vi "RTE PPL Test.vi"() -> ()   [LabVIEW 2020]
uses:
  PPL/HDH.ProjectBuilder.lvlibp/Class/PPL Class Test/PPL Class Test.lvclass
  PPL/HDH.ProjectBuilder.lvlibp/Class/Project Builder/Project Builder.lvclass
  PPL/HDH.ProjectBuilder.lvlibp/Class/PPL Class Test/PPL Class Test Data/PPL Class Test Data.lvclass
  PPL/HDH.ProjectBuilder.lvlibp/Interface/Action Interface/Action Interface.lvclass
  PPL/HDH.ProjectBuilder.lvlibp
panel:
  out "Load Success":string[](array[string])
  out "Load Failure":string[](array[string])
  out "Success?":bool
  in  "Run":bool
  in  "PPL Name in PPL folder (entire PPL folder if empty)":string
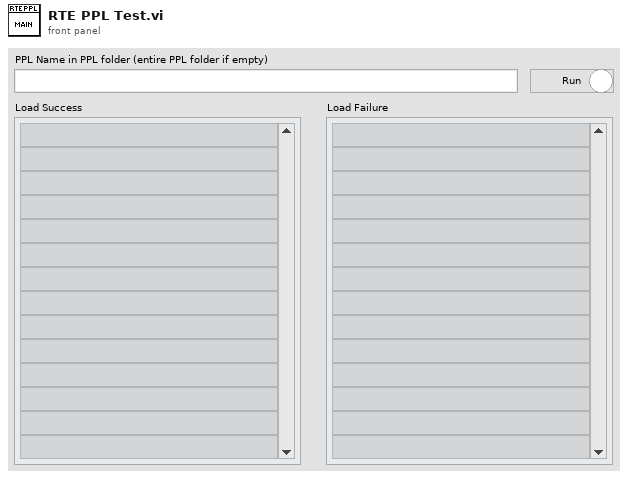
[diagram p1: front panel]
types:
  T1 = enum32{"Invalid", "Standard", "Closed", "Hidden", "Minimized", "Maximized"}
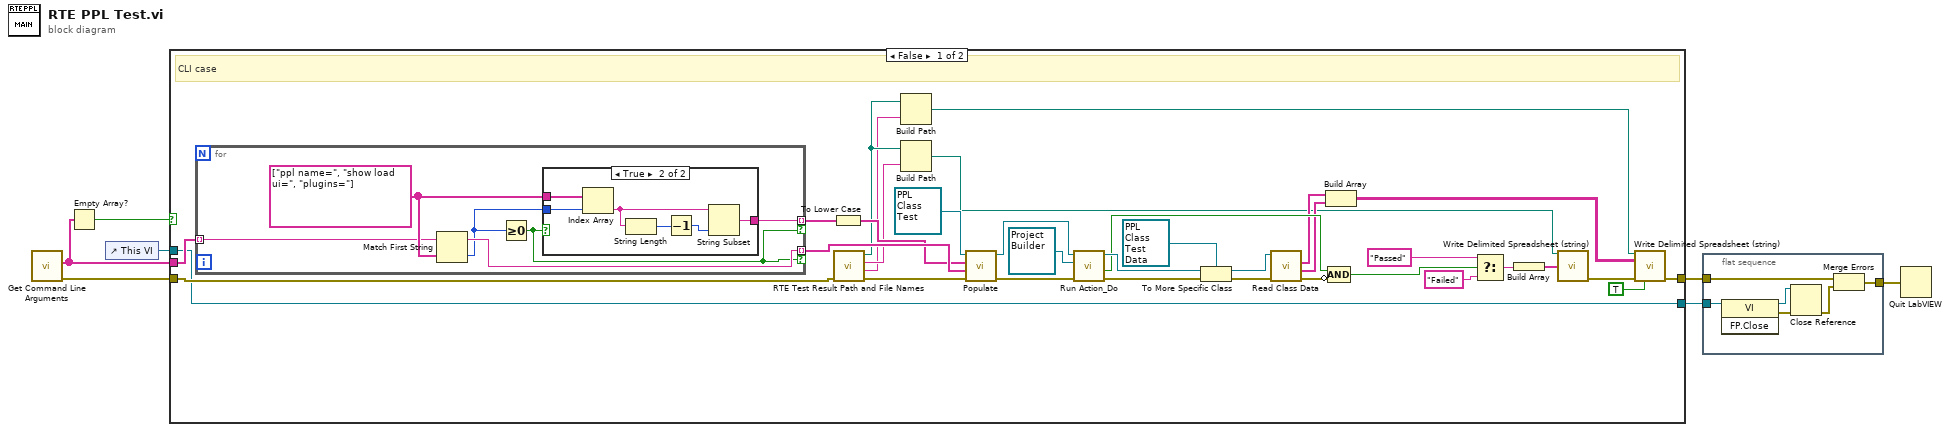
[diagram p0: block diagram]
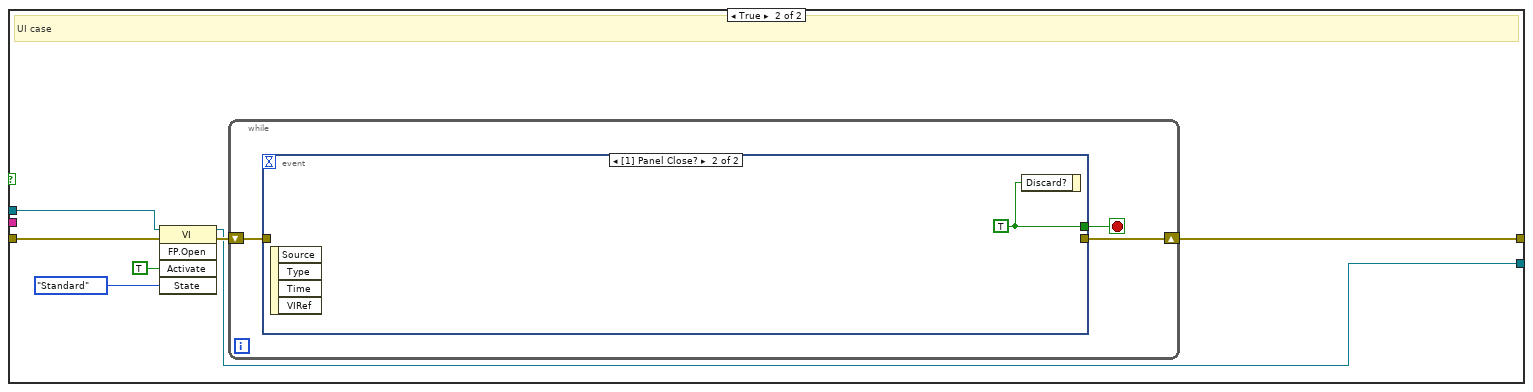
[diagram p3: hidden frame]
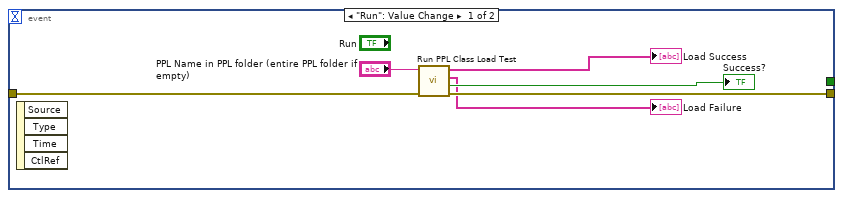
[diagram p4: hidden frame]
diagram:
  n1 = call <vilib>:"Get Command Line Arguments.vi"() -> ("error out"=w5:errorcluster, "arguments"=w6:string[])  [unwired: 9 in, 1 out]
  n2 = Empty Array?(array=w6) -> (empty?=w7:bool)
  n3 = control-ref of="This VI"() -> (w1:refnum<vi>)
  n4 = case shown="False" w7 {
    tunnel: w6 -> [w41 _]
    tunnel: [w10 w60] -> w4
    tunnel: w5 -> [w25 w55]
    tunnel: [w8 w54] -> w2
    tunnel: w1 -> [w8 w59]
    frame False {
      # "CLI case"
      n5 = for {
        tunnel: w41 -> [w45] mode=indexing
        tunnel: [w46] -> w38 mode=indexing if=w42
        tunnel: [w44] -> w39 mode=indexing if=w42
        w47 = string[] ["ppl name=", "show load ui=", "plugins="] ("string array")
        n6 = Match First String(2:w47, 3:w45) -> (0:w43:i32, 1:w46:string)
        n7 = Greater Or Equal To 0?(x=w43) -> (x >= 0?=w42:bool)
        n8 = case shown="True" w42 {
          tunnel: w47 -> [_ w53]
          tunnel: [_ w49] -> w44
          tunnel: w43 -> [_ w48]
          frame False {
          }
          frame True {
            n9 = Index Array(array=w53, index=w48) -> (element=w52:string)
            n10 = String Length(string=w52) -> (length=w51:i32)
            n11 = Decrement(x=w51) -> (x-1=w50:i32)
            n12 = String Subset(string=w52, length (rest)=w50) -> (substring=w49:string)  [unwired: 1 in]
          }
        }
      }
      n13 = To Lower Case(string=w39) -> (all lower case string=w37:string[])
      n14 = call "RTE Test Result Path and File Names.vi"("error in (no error)"=w25) -> ("error out"=w26:errorcluster, "PPL Test_Strings.txt"=w13:string, "PPL Test_Status.txt"=w16:string, "HDH\\ProjectBuilder\\temp path"=w14:path)  [unwired: 7 in]
      n15 = Build Path(base path=w14, name or relative path=w13) -> (appended path=w12:path)
      n16 = Build Path(base path=w14, name or relative path=w16) -> (appended path=w15:path)
      n17 = call "Populate.vi"("error in (no error)"=w26, "Values"=w38, "Names"=w37, "Action Interface in"=refnum<class "PPL Class Test.lvclass"> refnum ("HDH.ProjectBuilder.lvlibp:PPL Class Test.lvclass")) -> ("error out"=w34:errorcluster, "Action Interface out"=w36:refnum<class "PPL Class Test.lvclass">)  [unwired: 5 in, 1 out]
      n18 = call-dynamic "Run Action_Do.vi"("error in (no error)"=w34, "Project Builder in"=refnum<class "Project Builder.lvclass"> refnum, "PPL Class Test"=w36) -> ("error out"=w31:errorcluster, "Success?"=w28:bool, "Report"=w33:refnum<class "Report Data.lvclass">)  [unwired: 6 in]
      n19 = To More Specific Class(target class=refnum<class "PPL Class Test Data.lvclass"> refnum ("HDH.ProjectBuilder.lvlibp:PPL Class Test Data.lvclass"), reference=w33, error in=w31) -> (specific class reference=w30:refnum<class "PPL Class Test Data.lvclass">, error out=w29:errorcluster)
      n20 = call "Read Class Data.vi"("error in (no error)"=w29, "PPL Class Test Data in"=w30) -> ("error out"=w27:errorcluster, "Load Failure"=w23:string[], "Load Success"=w24:string[])  [unwired: 6 in, 1 out]
      n21 = Build Array(w24, w23) -> (w22:string[][])
      n22 = Compound Arithmetic op=AND(w28, invert w27) -> (w21:bool)
      n23 = Select(t="Passed" ("y"), s=w21, f="Failed" ("y")) -> (s? t:f=w18:string)
      n24 = Build Array(w18) -> (w17:string[])
      n25 = call <vilib>:"Write Delimited Spreadsheet (string).vi"("file path (dialog if empty)"=w15, "1D data"=w17) -> ("error out"=w11:errorcluster)  [unwired: 12 in, 1 out]
      n26 = call <vilib>:"Write Delimited Spreadsheet (string).vi"("file path (dialog if empty)"=w12, "2D data"=w22, "error in (no error)"=w11, "transpose? (no:F)"=TRUE) -> ("error out"=w10:errorcluster)  [unwired: 10 in, 1 out]
    }
    frame True {
      # "UI case"
      n27 = invoke class="VI" method="FP.Open"(reference=w59, error in=w55, "Activate"=TRUE, "State"=T1."Standard") -> (reference out=w54:refnum<vi>, error out=w56:errorcluster)  [unwired: 1 in, 3 out]
      n28 = while {
        shift-right: [w63] -> w60
        shift-left: w56 -> [w62]
        stop <- w61 stop-if-true
        n29 = event shown="[1] Panel Close?" {
          selector: _ -> [_ _]
          dyn-events: _ -> [_ _]
          timeout: _ -> [_ _]
          tunnel: [w69 _] -> w63
          tunnel: w62 -> [w68 _]
          tunnel: [_ w70] -> w61
          event "Run": Value Change {
            n30 = event-data() -> ()  [unwired: 1 in, 4 out]
            n31 = call "Run PPL Class Load Test.vi"("error in"=w68, "PPL Name in PPL folder (entire PPL folder if empty)"="PPL Name in PPL folder (entire PPL folder if empty)") -> ("error out"=w69:errorcluster, "Success?"=→"Success?":bool, "Load Failure"=→"Load Failure":string[], "Load Success"=→"Load Success":string[])  [unwired: 6 in]
          }
          event Panel Close? {
            w70 = TRUE
            n32 = event-data() -> ()  [unwired: 1 in, 4 out]
            n33 = event-data("Discard?"=w70) -> ()  [unwired: 1 in, 1 out]
          }
        }
      }
    }
  }
  n34 = flat-sequence {
    tunnel: w4 -> [w73]
    tunnel: [w72] -> w3
    tunnel: w2 -> [w71]
    frame #0 {
      n35 = invoke class="VI" method="FP.Close"(reference=w71) -> (reference out=w75:refnum<vi>, error out=w76:errorcluster)  [unwired: 2 in, 1 out]
      n36 = Close Reference(reference=w75, error in (no error)=w76) -> (error out=w74:errorcluster)
      n37 = Merge Errors(w73, w74) -> (w72:errorcluster)
    }
  }
  n38 = Quit LabVIEW(quit? (T)=w3) -> ()
